vi "Encode_UInt32.vi"(1 "UInt32":u32[](array[numeric])) -> (0 "Little Endian":u8[](array[numeric]))   [LabVIEW 2015, in "navX Library v3.lvlib" / "navX Registry Cache.lvclass"]
uses:
  navX Registry Cache.lvclass
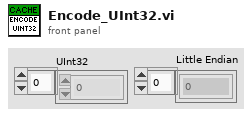
[diagram p1: front panel]
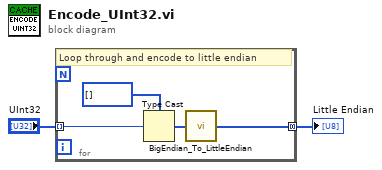
[diagram p0: block diagram]
diagram:
  n1 = for {
    tunnel: "UInt32" -> [w5] mode=indexing
    tunnel: [w3] -> w1 mode=concatenating
    # "Loop through and encode to little endian"
    n2 = Type Cast(type=u8[] [], x=w5) -> (*(type *) &x=w4:u8[])
    n3 = call "BigEndian_To_LittleEndian.vi"("Big Endian"=w4) -> ("Little Endian"=w3:u8[])
  }
  "Little Endian" <- w1
